vi "Temperature Device (Read).vi"(6 "ISOBUS address":T11=-1 caption="ISOBUS address (-1)", 8 "error in":errorcluster, 11 "Mercury Reference In":T12) -> (0 "error out":errorcluster, 2 "Device Details":T2, 3 "Mercury Reference Out":T12, 4 "Valid?":T1)   [LabVIEW 2016, in "Mercury iXX.lvlib" / "Temperature.lvlib"]
doc: "Read the current device configuration for the selected device."
uses:
  Temperature.lvlib
  Controls/Mercury Reference.ctl
  Controls/Comms Transport Layer.ctl
  Private/Controls/Query Dynamic Reference.ctl
  Controls/ISOBus Address.ctl
  Controls/Temperature Device (Read).ctl
  Controls/Manufacturing Data.ctl
  Controls/Temperature Sensor Type.ctl
  Controls/Excitation Cluster.ctl
  Controls/Excitation Type.ctl
  Controls/Calibration Cluster.ctl
  Controls/Calibration Interpolation.ctl
  Controls/Loop Cluster.ctl
  Controls/Temperature Signals Cluster.ctl
  Controls/Is Valid LED.ctl
  Private/Controls/Command Verbs.ctl
  Mercury iXX.lvlib
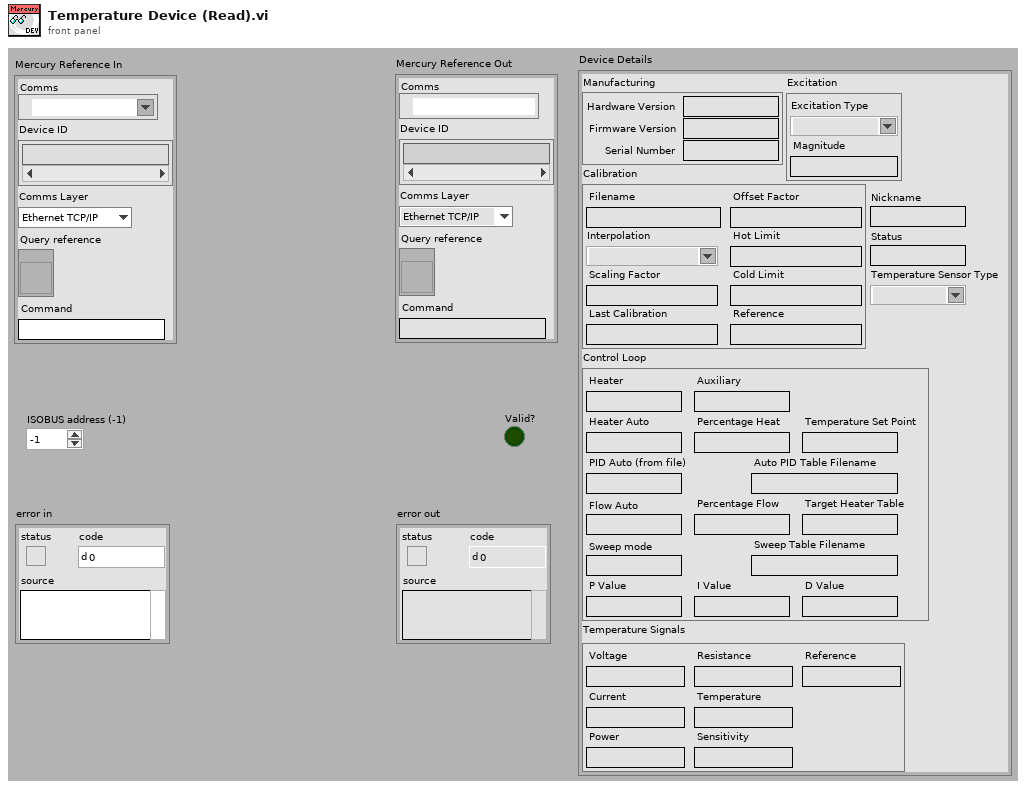
[diagram p1: front panel]
types:
  T1 = typedef "Mercury iXX.lvlib/Is Valid LED.ctl" = bool
  T2 = typedef "Mercury iXX.lvlib/Temperature.lvlib/Temperature Device (Read).ctl" = cluster{"Manufacturing":T3, "Temperature Sensor Type":T4, "Excitation":T5, "Calibration":T7, "Control Loop":T9, "Temperature Signals":T10, "Nickname":string, "Status":string}
  T3 = typedef "Mercury iXX.lvlib/Manufacturing Data.ctl" = cluster{"Hardware Version":string, "Firmware Version":string, "Serial Number":string}
  T4 = typedef "Mercury iXX.lvlib/Temperature.lvlib/Temperature Sensor Type.ctl" = string
  T5 = typedef "Mercury iXX.lvlib/Temperature.lvlib/Excitation Cluster.ctl" = cluster{"Excitation Type":T6, "Magnitude":string}
  T6 = typedef "Mercury iXX.lvlib/Temperature.lvlib/Excitation Type.ctl" = string
  T7 = typedef "Mercury iXX.lvlib/Temperature.lvlib/Calibration Cluster.ctl" = cluster{"Filename":string, "Interpolation":T8, "Scaling Factor":string, "Offset Factor":string, "Hot Limit":string, "Cold Limit":string, "Last Calibration":string, "Reference":string}
  T8 = typedef "Mercury iXX.lvlib/Temperature.lvlib/Calibration Interpolation.ctl" = string
  T9 = typedef "Mercury iXX.lvlib/Temperature.lvlib/Loop Cluster.ctl" = cluster{"Heater":string, "Auxiliary":string, "Heater Auto":string, "Percentage Heat":string, "Temperature Set Point":string, "PID Auto (from file)":string, "P Value":string, "I Value":string, "D Value":string, "Auto PID Table Filename":string, "Flow Auto":string, "Target Heater Table":string, "Sweep mode":string, "Sweep Table Filename":string, "Percentage Flow":string}
  T10 = typedef "Mercury iXX.lvlib/Temperature.lvlib/Temperature Signals Cluster.ctl" = cluster{"Voltage":string, "Current":string, "Power":string, "Resistance":string, "Temperature":string, "Sensitivity":string, "Reference":string}
  T11 = typedef "Mercury iXX.lvlib/ISOBus Address.ctl" = i32
  T12 = typedef "Mercury iXX.lvlib/Mercury Reference.ctl" = cluster{"Comms":refnum<visa-resource-name>, "Device ID":string[], "Comms Layer":T13, "Command":string, "Query reference":T14}
  T13 = typedef "Mercury iXX.lvlib/Comms Transport Layer.ctl" = enum16{"Ethernet TCP/IP", "USB", "ISOBus - RS-232", "GPIB"}
  T14 = typedef "Mercury iXX.lvlib/Query Dynamic Reference.ctl" = refnum<vi>
  T15 = typedef "Mercury iXX.lvlib/Command Verbs.ctl" = string
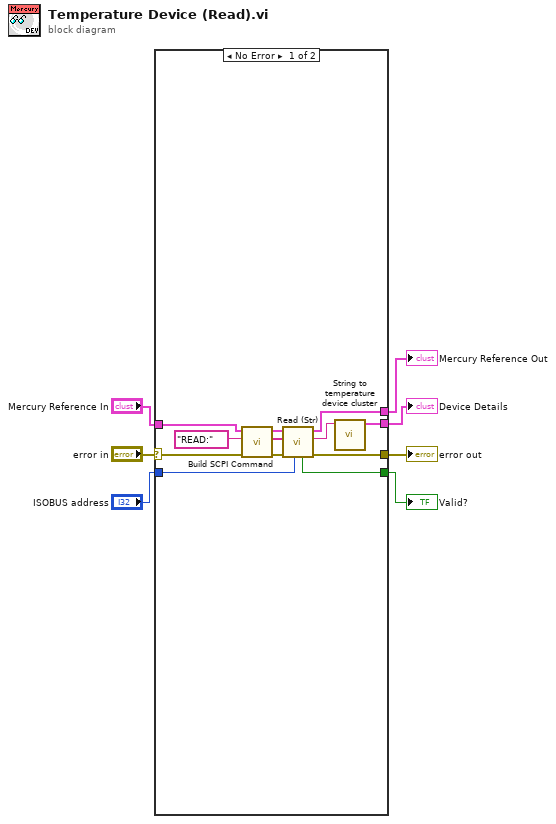
[diagram p0: block diagram]
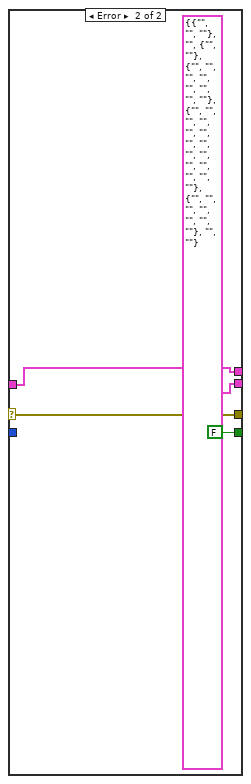
[diagram p2: hidden frame]
diagram:
  n1 = case shown="No Error" "error in" {
    selector: "error in" -> [w8 w23]
    tunnel: "Mercury Reference In" -> [w13 w21]
    tunnel: [w11 w23] -> w6
    tunnel: [w12 w21] -> w5
    tunnel: "ISOBUS address" -> [w9 _]
    tunnel: [w10 T1 FALSE ("Valid?")] -> w3
    tunnel: [w19 T2 {"Manufacturing"={"Hardware Version"="", "Firmware Version"="", "Serial Number"=""}, "Temperature Sensor Type"="", "Excitation"={"Excitation Type"="", "Magnitude"=""}, "Calibration"={"Filename"="", "Interpolation"="", "Scaling Factor"="", "Offset Factor"="", "Hot Limit"="", "Cold Limit"="", "Last Calibration"="", "Reference"=""}, "Control Loop"={"Heater"="", "Auxiliary"="", "Heater Auto"="", "Percentage Heat"="", "Temperature Set Point"="", "PID Auto (from file)"="", "P Value"="", "I Value"="", "D Value"="", "Auto PID Table Filename"="", "Flow Auto"="", "Target Heater Table"="", "Sweep mode"="", "Sweep Table Filename"="", "Percentage Flow"=""}, "Temperature Signals"={"Voltage"="", "Current"="", "Power"="", "Resistance"="", "Temperature"="", "Sensitivity"="", "Reference"=""}, "Nickname"="", "Status"=""} ("Temperature Device Settings")] -> w2
    frame No Error {
      n2 = call "Build SCPI Command.vi"("error in"=w8, "Verb"=T15 "READ:", "Mercury Reference In"=w13) -> ("error out"=w18:errorcluster, "SCPI Message(s)"=w15:string[], "Mercury Reference Out"=w16:T12)  [unwired: 1 in, 5 out]
      n3 = call "Read (Str).vi"("ISOBUS address"=w9, "error in"=w18, "SCPI Message(s)"=w15, "Mercury Reference In"=w16) -> ("error out"=w11:errorcluster, "Response"=w14:string, "Mercury Reference Out"=w12:T12, "Valid?"=w10:T1)  [unwired: 4 out]
      n4 = call "String to temperature device cluster.vi"("Temp Device Details"=w14) -> ("Temperature Device Settings"=w19:T2)  [unwired: 1 in, 9 out]
    }
    frame Error {
    }
  }
  "Mercury Reference Out" <- w5
  "error out" <- w6
  "Device Details" <- w2
  "Valid?" <- w3
